vi "校准记录.vi"(8 "error in (no error)":errorcluster, 9 "曲线模型":T1={"标液浓度1"=0.0, "测量吸光度1"=0.0, "样品1启用"=FALSE, "标液浓度2"=0.0, "测量吸光度2"=0.0, "样品2启用"=FALSE, "标液浓度3"=0.0, "测量吸光度3"=0.0, "样品3启用"=FALSE, "标液浓度4"=0.0, "测量吸光度4"=0.0, "样品4启用"=FALSE, "标液浓度5"=0.0, "测量吸光度5"=0.0, "样品5启用"=FALSE, "模型"=enum."线性", "精度"=4.0, "XY图"=[], "拟合公式"="", "r^2"=0.0, "标样一校准时间"=timestamp(0 s since 1904-01-01), "标样二校准时间"=timestamp(0 s since 1904-01-01), "标样三校准时间"=timestamp(0 s since 1904-01-01), "标样四校准时间"=timestamp(0 s since 1904-01-01), "标样五校准时间"=timestamp(0 s since 1904-01-01), "二次方程"={"c"=0.0, "x"=0.0, "x^2"=0.0}, "标定时间"=timestamp(0 s since 1904-01-01)} {"标定时间" format="%<%m/%d/%y %H:%M:%S>T"; "标样五校准时间" format="%<%m/%d/%y %H:%M:%S>T"; "标样四校准时间" format="%<%m/%d/%y %H:%M:%S>T"; "标样三校准时间" format="%<%m/%d/%y %H:%M:%S>T"; "标样二校准时间" format="%<%m/%d/%y %H:%M:%S>T"; "标样一校准时间" format="%<%m/%d/%y %H:%M:%S>T"; "r^2" format="%.7f"; "测量吸光度5" format="%#.6f"; "测量吸光度4" format="%#.6f"; "测量吸光度3" format="%#.6f"; "测量吸光度2" format="%#.6f"; "测量吸光度1" format="%#.6f"}, 10 "量程":enum16{"低量程", "高量程"}(ring), 11 "校准参数":u16(ring) items=["总氮"=2, "总磷"=1]) -> (0 "error out":errorcluster)   [LabVIEW 2016, in "斯坦道总磷.lvlib"]
uses:
  <vilib>/addons/database/Auxilliary.llb/DB Tools Column Info.ctl
  <vilib>/addons/database/Auxilliary.llb/DB Tools DataTypes.ctl
  <vilib>/addons/database/NI_Database_API.lvlib
  <vilib>/Utility/VariantDataType/VariantType.lvlib
panel:
  out "结果字符串":string
  in  "data in":T2
  # "校准时间"
  # "标液浓度"
  # "吸光值显示"
  # "标液一"
  # "标液二"
  # "标液三"
  # "零点"
  # "跨度"
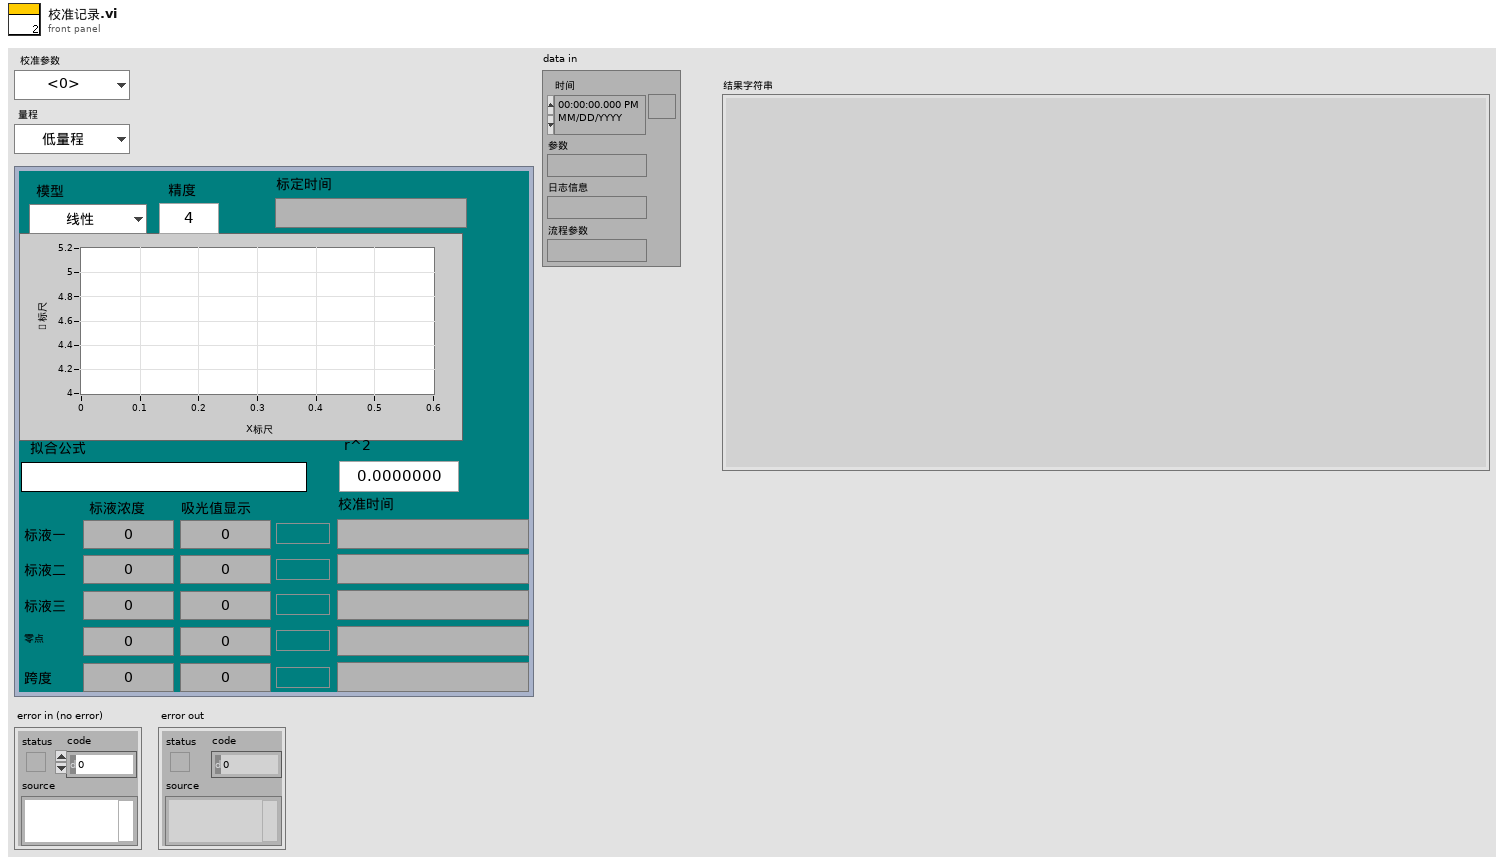
[diagram p1: front panel]
types:
  T1 = cluster{"标液浓度1":dbl, "测量吸光度1":dbl, "样品1启用":bool, "标液浓度2":dbl, "测量吸光度2":dbl, "样品2启用":bool, "标液浓度3":dbl, "测量吸光度3":dbl, "样品3启用":bool, "标液浓度4":dbl, "测量吸光度4":dbl, "样品4启用":bool, "标液浓度5":dbl, "测量吸光度5":dbl, "样品5启用":bool, "模型":enum32{"线性", "多项式"}, "精度":dbl, "XY图":cluster{"X Values":dbl[], "Y Values":dbl[]}[], "拟合公式":string, "r^2":dbl, "标样一校准时间":timestamp, "标样二校准时间":timestamp, "标样三校准时间":timestamp, "标样四校准时间":timestamp, "标样五校准时间":timestamp, "二次方程":cluster{"c":dbl, "x":dbl, "x^2":dbl}, "标定时间":timestamp}
  T2 = cluster{"时间":timestamp, "参数":string, "日志信息":string, "流程参数":string}
  T3 = typedef "NI_Database_API.lvlib/DB Tools Column Info.ctl" = cluster{"column name":string, "data type":T4, "size":i32, "allow null?":bool}
  T4 = typedef "NI_Database_API.lvlib/DB Tools DataTypes.ctl" = enum16{"String", "Long (I32)", "Single (SGL)", "Double (DBL)", "Date/Time", "Binary"}
  T5 = typedef "VariantType.lvlib/Type.ctl" = enum8{"Invalid Type", "Void", "I8", "I16", "I32", "I64", "U8", "U16", "U32", "U64", "Single Float", "Double Float", "Extended Float", "Single Complex", "Double Complex", "Extended Complex", "Enum U8", "Enum U16", "Enum U32", "Enum U64", "Single Float With Unit", "Double Float With Unit", "Extended Float With Unit", "Single Complex with Unit", "Double Complex with Unit", "Extended Complex with Unit", "Boolean", "String", "Path", "Picture", "Tag", "Array", "Cluster", "Variant", "LV Variant", "Waveform", "Timestamp", "Digital Waveform", "Digital Data", "ExpressData", "Refnum", "External Data", "VI", "Poly VI", "LabVIEW Class Instance", "Fixed Point"}
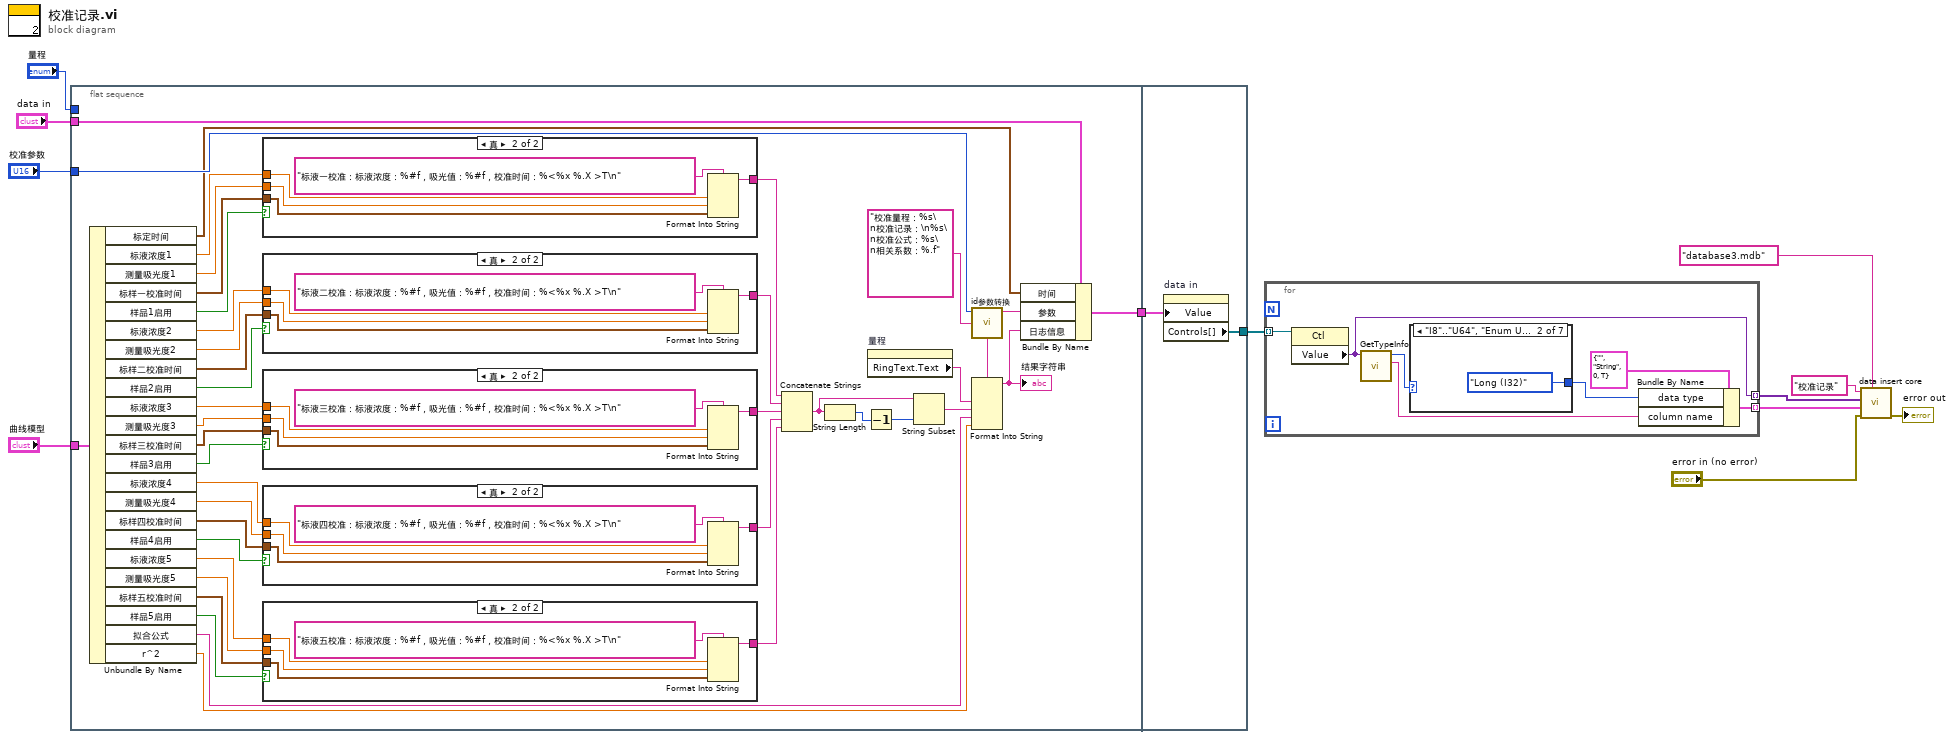
[diagram p0: block diagram]
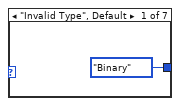
[diagram p7: hidden frame]
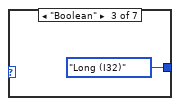
[diagram p8: hidden frame]
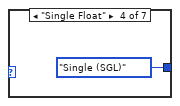
[diagram p9: hidden frame]
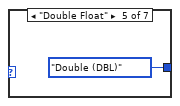
[diagram p10: hidden frame]
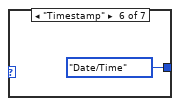
[diagram p11: hidden frame]
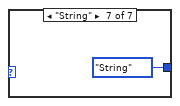
[diagram p12: hidden frame]
diagram:
  n1 = flat-sequence {
    tunnel: "校准参数" -> [w52]
    tunnel: "量程" -> [_]
    tunnel: "曲线模型" -> [w46]
    tunnel: "data in" -> [w51]
    tunnel: [w49] -> w1
    tunnel: [w79] -> w10
    tunnel: w1 -> [w78]
    frame #0 {
      n2 = Unbundle By Name(w46) -> ("标定时间"=w14:timestamp, "标液浓度1"=w44:dbl, "测量吸光度1"=w43:dbl, "标样一校准时间"=w42:timestamp, "样品1启用"=w45:bool, "标液浓度2"=w41:dbl, "测量吸光度2"=w40:dbl, "标样二校准时间"=w39:timestamp, "样品2启用"=w38:bool, "标液浓度3"=w37:dbl, "测量吸光度3"=w36:dbl, "标样三校准时间"=w35:timestamp, "样品3启用"=w34:bool, "标液浓度4"=w33:dbl, "测量吸光度4"=w32:dbl, "标样四校准时间"=w31:timestamp, "样品4启用"=w30:bool, "标液浓度5"=w29:dbl, "测量吸光度5"=w28:dbl, "标样五校准时间"=w27:timestamp, "样品5启用"=w26:bool, "拟合公式"=w20:string, "r^2"=w19:dbl)
      n3 = case shown="真" w45 {
        tunnel: w44 -> [_ w76]
        tunnel: w43 -> [_ w75]
        tunnel: w42 -> [_ w74]
        tunnel: [_ w73] -> w25
        frame False {
        }
        frame True {
          n4 = Format Into String(format string="标液一校准：标液浓度：%#f，吸光值：%#f，校准时间：%<%x %.X >T\n" ("格式字符串"), w76, w75, w74) -> (resulting string=w73:string)  [unwired: 2 in, 1 out]
        }
      }
      n5 = case shown="真" w38 {
        tunnel: w41 -> [_ w71]
        tunnel: w40 -> [_ w70]
        tunnel: w39 -> [_ w69]
        tunnel: [_ w68] -> w24
        frame False {
        }
        frame True {
          n6 = Format Into String(format string="标液二校准：标液浓度：%#f，吸光值：%#f，校准时间：%<%x %.X >T\n" ("格式字符串"), w71, w70, w69) -> (resulting string=w68:string)  [unwired: 2 in, 1 out]
        }
      }
      n7 = case shown="真" w34 {
        tunnel: w37 -> [_ w66]
        tunnel: w36 -> [_ w65]
        tunnel: w35 -> [_ w64]
        tunnel: [_ w63] -> w23
        frame False {
        }
        frame True {
          n8 = Format Into String(format string="标液三校准：标液浓度：%#f，吸光值：%#f，校准时间：%<%x %.X >T\n" ("格式字符串"), w66, w65, w64) -> (resulting string=w63:string)  [unwired: 2 in, 1 out]
        }
      }
      n9 = case shown="真" w30 {
        tunnel: w33 -> [_ w61]
        tunnel: w32 -> [_ w60]
        tunnel: w31 -> [_ w59]
        tunnel: [_ w58] -> w22
        frame False {
        }
        frame True {
          n10 = Format Into String(format string="标液四校准：标液浓度：%#f，吸光值：%#f，校准时间：%<%x %.X >T\n" ("格式字符串"), w61, w60, w59) -> (resulting string=w58:string)  [unwired: 2 in, 1 out]
        }
      }
      n11 = case shown="真" w26 {
        tunnel: w29 -> [_ w56]
        tunnel: w28 -> [_ w55]
        tunnel: w27 -> [_ w54]
        tunnel: [_ w53] -> w21
        frame False {
        }
        frame True {
          n12 = Format Into String(format string="标液五校准：标液浓度：%#f，吸光值：%#f，校准时间：%<%x %.X >T\n" ("格式字符串"), w56, w55, w54) -> (resulting string=w53:string)  [unwired: 2 in, 1 out]
        }
      }
      n13 = Concatenate Strings(w25, w24, w23, w22, w21) -> (w17:string)
      n14 = String Length(string=w17) -> (length=w16:i32)
      n15 = Decrement(x=w16) -> (x-1=w15:i32)
      n16 = property on="量程" class="Enum (严格)"() -> ("RingText.Text"=w13:string)  [unwired: 2 in, 2 out]
      n17 = String Subset(string=w17, length (rest)=w15) -> (substring=w18:string)  [unwired: 1 in]
      n18 = call "id参数转换.vi"("id"=w52) -> ("table输出"=w50:string)  [unwired: 9 in, 1 out]
      n19 = Format Into String(format string="校准量程：%s\n校准记录：\n%s\n校准公式：%s\n相关系数：%.f" ("格式字符串"), w13, w18, w20, w19) -> (resulting string=w48:string)  [unwired: 2 in, 1 out]
      "结果字符串" <- w48
      n20 = Bundle By Name(cluster=w51, "时间"=w14, "参数"=w50, "日志信息"=w48) -> (w49:T2)
    }
    frame #1 {
      n21 = property on="data in" class="Clust (严格)"("Value"=w78) -> ("Controls[]"=w79:refnum<vi>[])  [unwired: 2 in, 2 out]
    }
  }
  n22 = for {
    tunnel: w10 -> [w86] mode=indexing
    tunnel: [w81] -> w8 mode=indexing
    tunnel: [w82] -> w9 mode=indexing
    n23 = property class="Ctl"(reference=w86) -> ("Value"=w81:variant)  [unwired: 1 in, 2 out]
    n24 = call <vilib>:"GetTypeInfo.vi"("Variant"=w81) -> ("Name"=w80:string, "Type Enum"=w84:T5)  [unwired: 6 in, 3 out]
    n25 = case shown="\"I8\"..\"U64\", \"Enum U8\"..\"Enum U64\"" w84 {
      tunnel: [DB_Tools_DataTypes."Binary" ("data type") DB_Tools_DataTypes."Long (I32)" ("data type") DB_Tools_DataTypes."Long (I32)" ("data type") DB_Tools_DataTypes."Single (SGL)" ("data type") DB_Tools_DataTypes."Double (DBL)" ("data type") DB_Tools_DataTypes."Date/Time" ("data type") DB_Tools_DataTypes."String" ("data type")] -> w83
      frame "Invalid Type", Default {
      }
      frame "I8".."U64", "Enum U8".."Enum U64" {
      }
      frame "Boolean" {
      }
      frame "Single Float" {
      }
      frame "Double Float" {
      }
      frame "Timestamp" {
      }
      frame "String" {
      }
    }
    n26 = Bundle By Name(cluster=T3 {"column name"="", "data type"=enum."String", "size"=0, "allow null?"=TRUE} ("column information"), "data type"=w83, "column name"=w80) -> (w82:T3)
  }
  n27 = call "data insert core.vi"("database"="database3.mdb", "error in (no error)"="error in (no error)", "column information"=w9, "data"=w8, "table"="校准记录") -> ("error out"=→"error out":errorcluster)  [unwired: 6 in]
